vi "Write.vi"(8 "error in":errorcluster, 10 "Write":T1={"Data (dec)"=0, FALSE, "Index"="``", "Sub-Index"="\u0000", "Data-Size (in Byte)"=1} {"Data-Size (in Byte)" min=1 max=4 step=1 format="%x"; "Data (dec)" step=1}, 11 "ComPort In":refnum<visa-resource-name>="COM15") -> (0 "error out":errorcluster, 3 "ComPort Out":refnum<visa-resource-name>)   [LabVIEW 2021]
uses:
  <vilib>/Instr/_visa.llb/VISA Flush IO Buffer Mask.ctl
panel:
  out "return count":u32
  out "read buffer Processed":string
  out "Numeric Output":i32
  out "read buffer raw":string
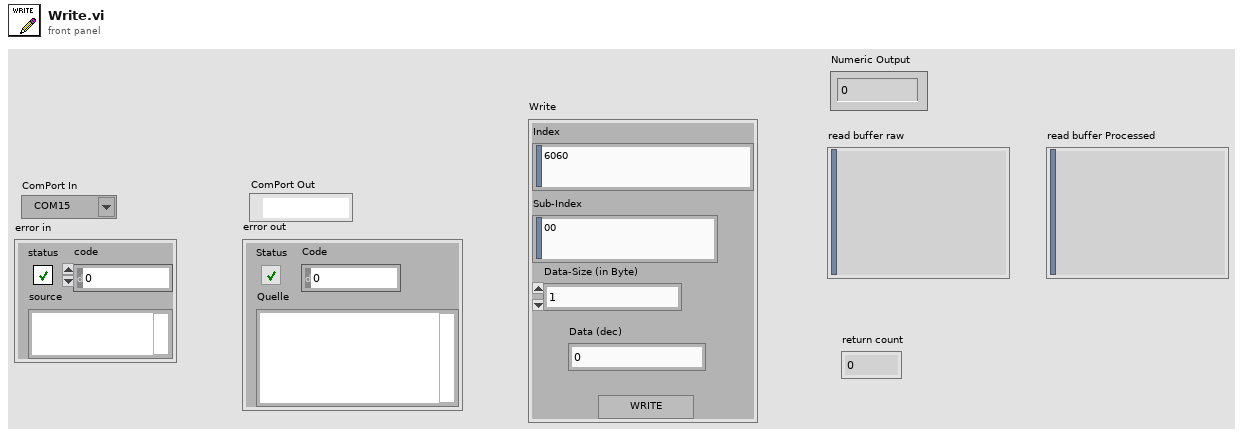
[diagram p1: front panel]
types:
  T1 = cluster{"Data (dec)":i32, bool, "Index":string, "Sub-Index":string, "Data-Size (in Byte)":u8}
  T2 = typedef "VISA Flush IO Buffer Mask.ctl" = u16
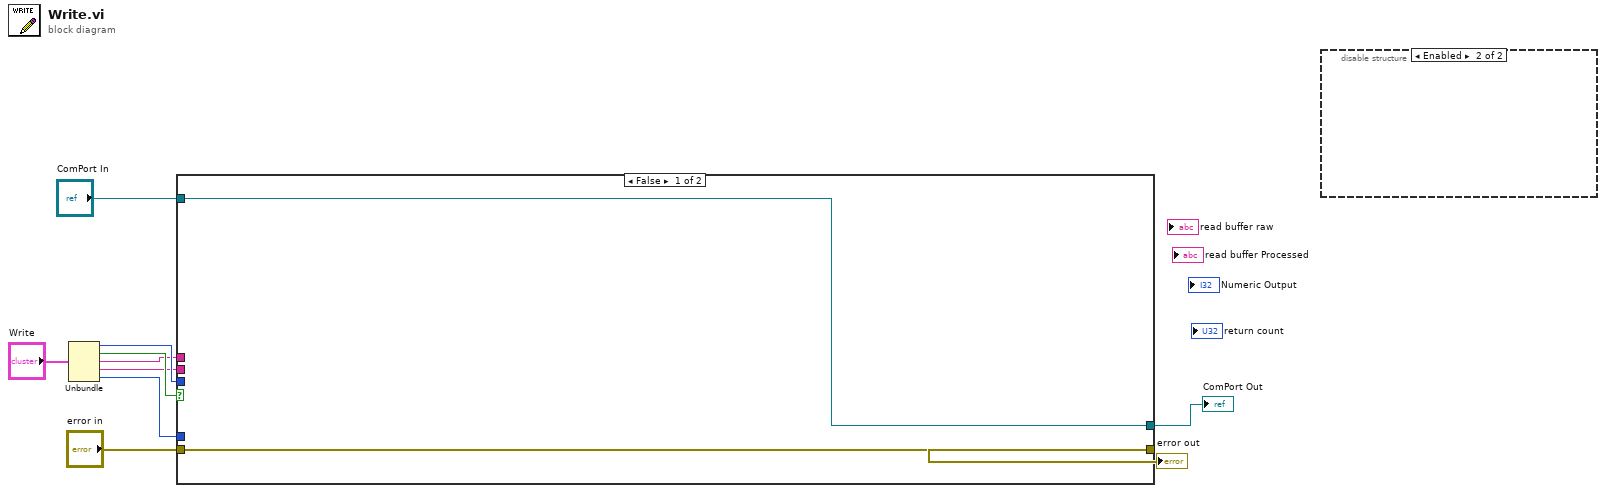
[diagram p0: block diagram]
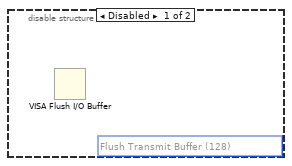
[diagram p2: hidden frame]
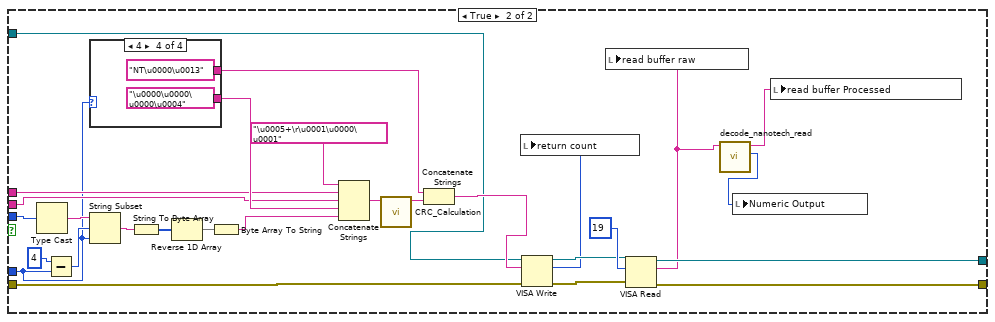
[diagram p3: hidden frame]
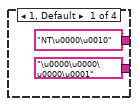
[diagram p4: hidden frame]
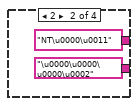
[diagram p5: hidden frame]
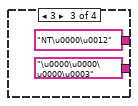
[diagram p6: hidden frame]
diagram:
  n1 = Unbundle("Write") -> ("Data (dec)"=w4:i32, w5:bool, "Index"=w2:string, "Sub-Index"=w1:string, "Data-Size (in Byte)"=w3:u8)
  n2 = case shown="False" w5 {
    tunnel: "ComPort In" -> [w12 w14]
    tunnel: "error in" -> [w11 w13]
    tunnel: [w12 w31] -> w10
    tunnel: [w11 w30] -> w9
    tunnel: w3 -> [_ w24]
    tunnel: w2 -> [_ w29]
    tunnel: w1 -> [_ w28]
    tunnel: w4 -> [_ w22]
    frame False {
    }
    frame True {
      n3 = Type Cast(x=w22) -> (*(type *) &x=w27:string)  [unwired: 1 in]
      n4 = Subtract(x=u8 4, y=w24) -> (x-y=w26:u8)
      n5 = case shown="4" w24 {
        tunnel: ["NT\u0000\u0010" ("Hexadecimal Input String 4") "NT\u0000\u0011" ("Hexadecimal Input String 4") "NT\u0000\u0012" ("Hexadecimal Input String 4") "NT\u0000\u0013" ("Hexadecimal Input String 4")] -> w39
        tunnel: ["\u0000\u0000\u0000\u0001" ("Hexadecimal Input String 4") "\u0000\u0000\u0000\u0002" ("Hexadecimal Input String 4") "\u0000\u0000\u0000\u0003" ("Hexadecimal Input String 4") "\u0000\u0000\u0000\u0004" ("Hexadecimal Input String 4")] -> w40
        frame 1, Default {
        }
        frame 2 {
        }
        frame 3 {
        }
        frame 4 {
        }
      }
      n6 = String Subset(string=w27, offset (0)=w26, length (rest)=w24) -> (substring=w23:string)
      n7 = String To Byte Array(string=w23) -> (unsigned byte array=w34:u8[])
      n8 = Reverse 1D Array(array=w34) -> (reversed array=w36:u8[])
      n9 = Byte Array To String(unsigned byte array=w36) -> (string=w37:string)
      n10 = Concatenate Strings("\u0005+\r\u0001\u0000\u0001" ("Hexadecimal Input String 4"), w29, w28, w40, w37) -> (w33:string)
      n11 = call "CRC_Calculation.vi"("CMD"=w33) -> ("CMD + CRC"=w32:string)  [unwired: 10 in]
      n12 = Concatenate Strings(w39, w32) -> (w19:string)
      n13 = VISA Write(VISA resource name=w14, write buffer=w19, error in (no error)=w13) -> (VISA resource name out=w21:refnum<visa-resource-name>, return count=w15:u32, error out=w20:errorcluster)
      n14 = local write "return count"(w15) -> ()
      n15 = VISA Read(VISA resource name=w21, byte count=u32 19, error in (no error)=w20) -> (VISA resource name out=w31:refnum<visa-resource-name>, read buffer=w18:string, error out=w30:errorcluster)  [unwired: 1 out]
      n16 = local write "read buffer raw"(w18) -> ()
      n17 = call "decode_nanotech_read.vi"("read buffer in"=w18) -> ("Numeric Output"=w17:i32, "read buffer out"=w16:string)  [unwired: 9 in]
      n18 = local write "Numeric Output"(w17) -> ()
      n19 = local write "read buffer Processed"(w16) -> ()
    }
  }
  "ComPort Out" <- w10
  "error out" <- w9
  n20 = disable-structure shown="Enabled" {
    frame Disabled {
      (unwired) T2 128 items=["Flush Receive Buffer"=16, "Write Transmit Buffer to Device"=32, "Flush Receive Buffer (No I/O)"=64, "Flush Transmit Buffer"=128] ("Mask")
      n21 = VISA Flush I/O Buffer() -> ()  [unwired: 3 in, 2 out]
    }
    frame Enabled {
    }
  }
